vi "Get CLI Version.vi"(8 "error in":errorcluster) -> (0 "error out":errorcluster, 3 "full version string":string)   [LabVIEW 2014, in "NIPM_API.lvlib"]
doc: "Returns the current version of the NIPKG command-line interface (CLI)"
uses:
  NIPM_API.lvlib
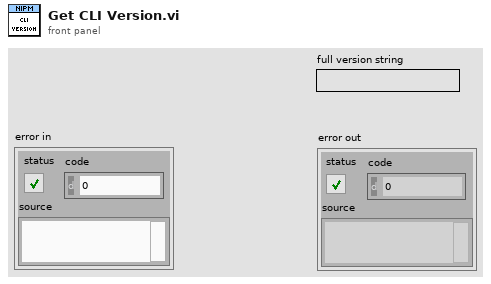
[diagram p1: front panel]
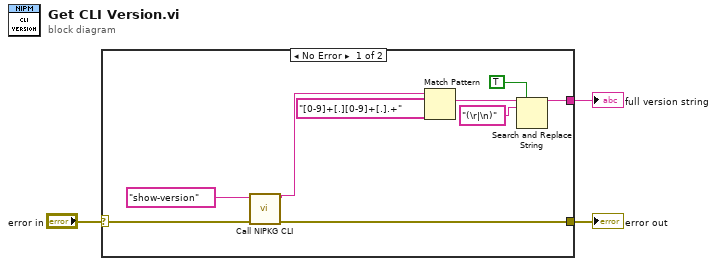
[diagram p0: block diagram]
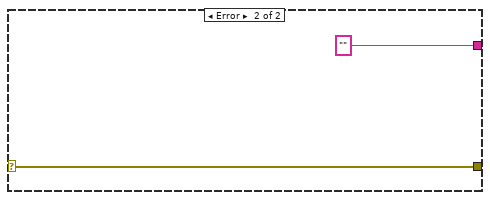
[diagram p2: hidden frame]
diagram:
  n1 = case shown="No Error" "error in" {
    selector: "error in" -> [w4 w14]
    tunnel: [w8 "" ("standard output")] -> w2
    tunnel: [w5 w14] -> w1
    frame No Error {
      n2 = call "Call NIPKG CLI.vi"("error in (no error)"=w4, "command"="show-version" ("format string")) -> ("error out"=w5:errorcluster, "command line standard output"=w6:string)  [unwired: 8 in]
      n3 = Match Pattern(string=w6, regular expression="[0-9]+[.][0-9]+[.].+") -> (match substring=w11:string)  [unwired: 1 in, 3 out]
      n4 = Search and Replace String(replace all?=TRUE ("replace all? (F)"), input string=w11, search string="(\r|\n)") -> (result string=w8:string)  [unwired: 5 in, 3 out]
    }
    frame Error {
    }
  }
  "error out" <- w1
  "full version string" <- w2
